vi "Get Test Members.vi"(7 "application reference (local)":refnum<vi>, 8 "error in (no error)":errorcluster, 10 "Test Class Path":path) -> (0 "error out":errorcluster, 2 "Test Members":path[](array[path]))   [LabVIEW 2011, in "VITesterUtilities.lvlib"]
uses:
  Libraries/VITesterUtilities.lvlib
  <userlib>/_OpenG.lib/array/array.llb/Remove Duplicates from 1D Array (Path)__ogtk.vi
  <userlib>/_OpenG.lib/array/array.llb/Conditional Auto-Indexing Tunnel (Path)__ogtk.vi
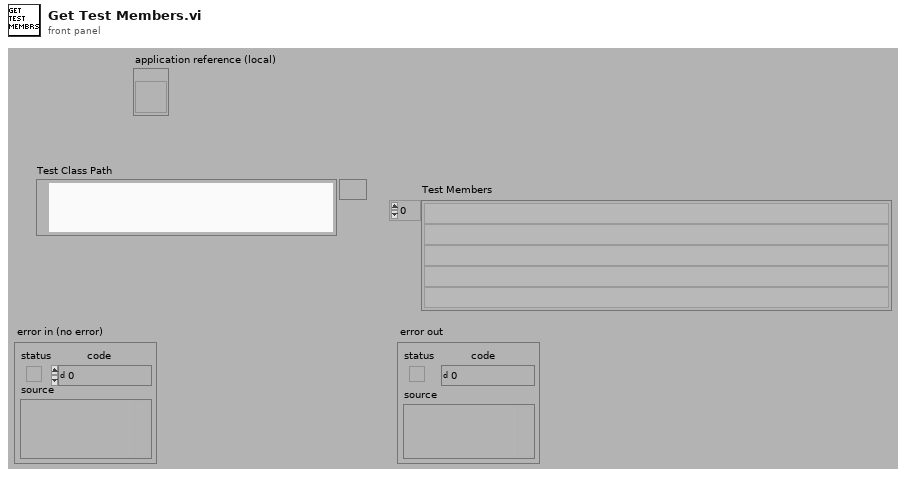
[diagram p1: front panel]
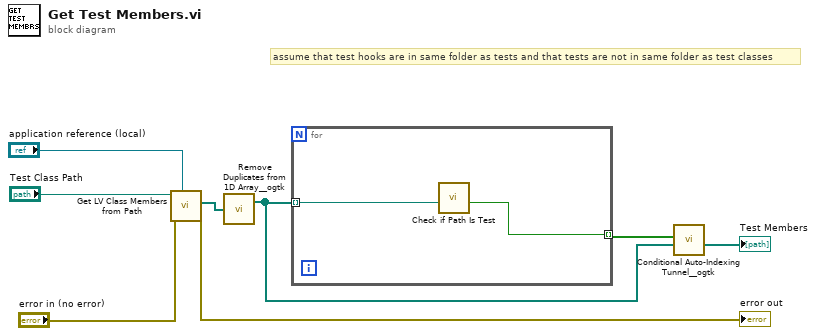
[diagram p0: block diagram]
diagram:
  # "assume that test hooks are in same folder as tests and that tests are not in same folder as test classes"
  n1 = call "Get LV Class Members from Path.vi"("application reference (local)"="application reference (local)", "error in (no error)"="error in (no error)", "Class Path"="Test Class Path") -> ("error out"=→"error out":errorcluster, "LV Class Members"=w3:path[])  [unwired: 7 in]
  n2 = call-poly <userlib>:"Remove Duplicates from 1D Array__ogtk.vi"("Input Array"=w3) -> ("Output Array"=w1:path[])  [unwired: 1 out]
  n3 = for {
    tunnel: [w9] -> w8 mode=indexing
    tunnel: w1 -> [w10] mode=indexing
    n4 = call "Check if Path Is Test.vi"("Path"=w10) -> ("IsTest?"=w9:bool)  [unwired: 10 in]
  }
  n5 = call-poly <userlib>:"Conditional Auto-Indexing Tunnel__ogtk.vi"("Array in"=w1, "Elements to keep"=w8) -> ("Filtered Array out"=→"Test Members":path[])  [unwired: 5 in]
